vi "Create Digital Waveform.vi"(8 "error in (no error)":errorcluster, 9 "Type (0: dwfSine)":i32(ring) items=["dwfSine", "dwfPhasedSine", "dwfNoise", "dwfUSASI", "dwfSquare", "dwfRamp", "dwfArb", "dwfChirp", "dwfMultiTone", "dwfIMD", "dwfConstant", "dwfCount", "dwfRotate", "dwfStair", "dwfJTest", "dwfPolarity", "dwfMLS", "dwfLogSine"], 10 "Channel (0: A)":i32(ring) items=["A", "B"], 11 "VISA resource name":refnum<visa-resource-name>) -> (0 "error out":errorcluster, 2 "Waveform Channel ID":i32, 3 "VISA resource name out":refnum<visa-resource-name>)   [LabVIEW 2014, in "Stanford Research SR1.lvlib"]
doc: "Adds a waveformof the specified type to the digital generator. The value returned is the ID of the new waveform."
uses:
  Stanford Research SR1.lvlib
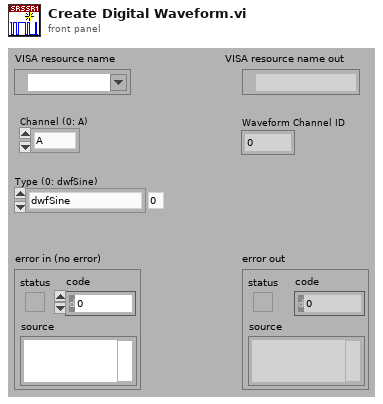
[diagram p1: front panel]
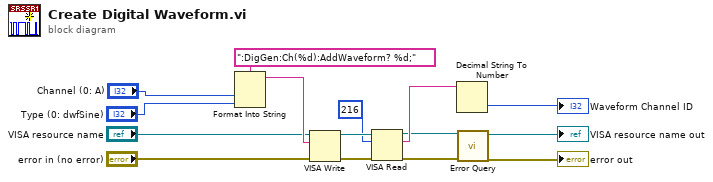
[diagram p0: block diagram]
diagram:
  n1 = Format Into String(format string=":DigGen:Ch(%d):AddWaveform? %d;", "Channel (0: A)", "Type (0: dwfSine)") -> (resulting string=w14:string)  [unwired: 2 in, 1 out]
  n2 = VISA Write(VISA resource name="VISA resource name", write buffer=w14, error in (no error)="error in (no error)") -> (VISA resource name out=w7:refnum<visa-resource-name>, error out=w6:errorcluster)  [unwired: 1 out]
  n3 = VISA Read(VISA resource name=w7, byte count=u32 216, error in (no error)=w6) -> (VISA resource name out=w1:refnum<visa-resource-name>, read buffer=w4:string, error out=w2:errorcluster)  [unwired: 1 out]
  n4 = Decimal String To Number(string=w4) -> (number=→"Waveform Channel ID":i32)  [unwired: 2 in, 1 out]
  n5 = call "Error Query.vi"("error in (no error)"=w2, "VISA resource name"=w1) -> ("error out"=→"error out":errorcluster, "VISA resource name out"=→"VISA resource name out":refnum<visa-resource-name>)  [unwired: 6 in, 2 out]
